vi "swmm_modify_setting.vi"(3 "error in":errorcluster, 4 "new_setting":dbl, 5 "id":string) -> (0 "error out":errorcluster, 1 "value":i32)   [LabVIEW 2014]
uses:
  swmm5.dll
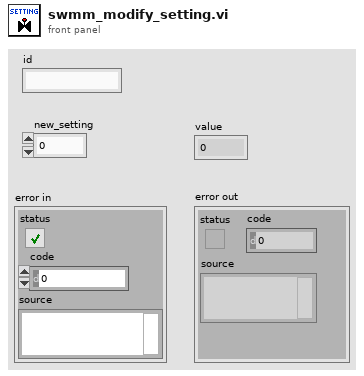
[diagram p1: front panel]
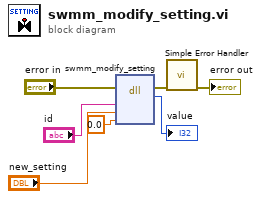
[diagram p0: block diagram]
diagram:
  n1 = dll-call lib="PTH2zabs CUsers\nandres riañoDropboxProyecto AguasSoftwareMatSWMMMatSWMM 5.1.009LabVIEW modulex64\tswmm5.dll" fn="swmm_modify_setting"(error in="error in", "id"="id", "new_setting"="new_setting", "tstep"=0.0) -> (error out=w2:errorcluster, "return type"=→"value":i32)  [unwired: 5 in, 1 out]
  n2 = call <vilib>:"Simple Error Handler.vi"("error in (no error)"=w2) -> ("error out"=→"error out":errorcluster)  [unwired: 4 in, 4 out]
